vi "WinCI Get Advanced Command Options.vi"(7 "advanced options in":variant, 8 "error in (no error)":errorcluster, 10 "command":T1 items=["GET", "CHECKOUT", "CHECKIN", "UNDOCHECKOUT", "ADD", "REMOVE", "COMPARE", "FILEHISTORY", "FILEPROPERTIES", "CONFIGOPTIONS"], 11 "source control reference in":T2) -> (0 "error out":errorcluster, 1 "dialog box cancelled?":bool, 2 "status message":string, 3 "source control reference out":T2, 5 "advanced options out":variant)   [LabVIEW 2020, in "NI_SCC_WinCI.lvlib"]
uses:
  <vilib>/SourceControl/Providers/WinCI/NI_SCC_WinCI.lvlib
  <vilib>/SourceControl/sccapi/SCCAPI Refnum.ctl
  <vilib>/SourceControl/sccapi/SCCAPI Command.ctl
  <vilib>/SourceControl/support/SCCSup Message Strings GLBL.vi
  <vilib>/SourceControl/sccapi/NI_SCC.lvlib
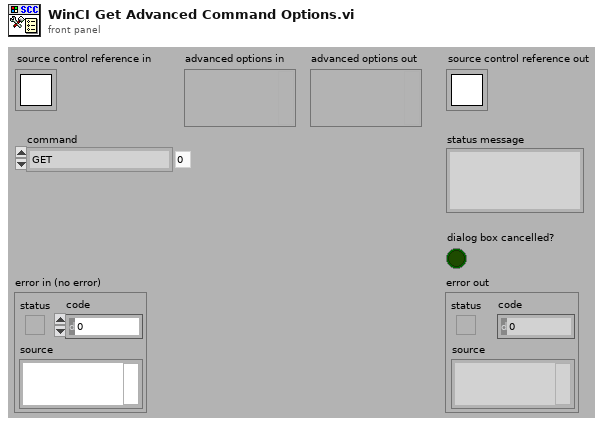
[diagram p1: front panel]
types:
  T1 = typedef "NI_SCC.lvlib/SCCAPI Command.ctl" = i32
  T2 = typedef "NI_SCC.lvlib/SCCAPI Refnum.ctl" = refnum<k1>
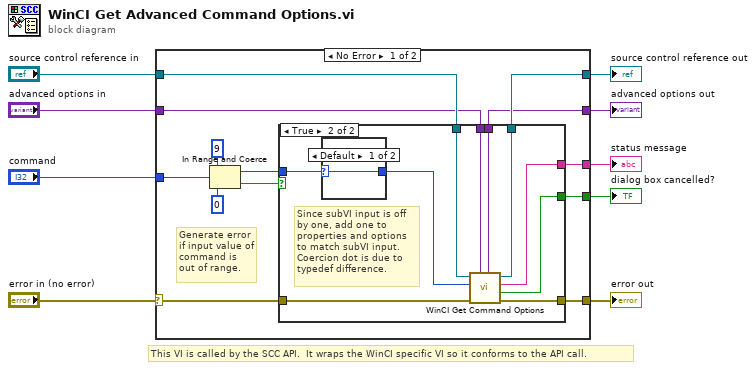
[diagram p0: block diagram]
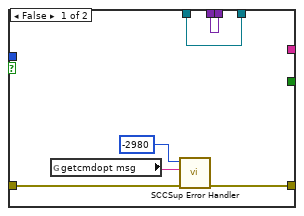
[diagram p2: hidden frame]
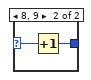
[diagram p3: hidden frame]
diagram:
  # "This VI is called by the SCC API.  It wraps the WinCI specific VI so it conforms to the API call."
  n1 = case shown="No Error" "error in (no error)" {
    selector: "error in (no error)" -> [w19 w44]
    tunnel: [w18 w44] -> w8
    tunnel: "source control reference in" -> [w17 w43]
    tunnel: [w15 _] -> w6
    tunnel: "command" -> [w20 _]
    tunnel: [w14 _] -> w4
    tunnel: [w16 w43] -> w3
    tunnel: [w12 w42] -> w2
    tunnel: "advanced options in" -> [w11 w42]
    frame No Error {
      # "Generate error if input value of command is out of range."
      n2 = In Range and Coerce(upper limit=9, x=w20, lower limit=0) -> (coerced(x)=w13:T1, In Range?=w10:bool)
      n3 = case shown="True" w10 {
        tunnel: w19 -> [w25 w29]
        tunnel: [w24 w30] -> w18
        tunnel: w17 -> [w27 w34]
        tunnel: [w27 w35] -> w16
        tunnel: [_ w32] -> w15
        tunnel: [_ w31] -> w14
        tunnel: w13 -> [_ w38]
        tunnel: [w28 w36] -> w12
        tunnel: w11 -> [w28 w37]
        frame False {
          n4 = global read "SCCSup Message Strings GLBL.vi" "getcmdopt msg"() -> (w26:string)
          n5 = call <vilib>:"SCCSup Error Handler.vi"("error in (no error)"=w25, "operation message"=w26, "scc error code"=-2980 ("error code")) -> ("error out"=w24:errorcluster)  [unwired: 1 in, 7 out]
        }
        frame True {
          # "Since subVI input is off by one, add one to properties and options to match subVI input.  Coercion dot is due to typedef difference."
          n6 = case shown="Default" w38 {
            selector: w38 -> [w39 w41]
            tunnel: [w39 w40] -> w33
            frame Default {
            }
            frame 8, 9 {
              n7 = Increment(x=w41) -> (x+1=w40:T1)
            }
          }
          n8 = call <vilib>:"WinCI Get Command Options.vi"("advanced options in"=w37, "error in (no error)"=w29, "interface command"=w33, "source control reference in"=w34) -> ("error out"=w30:errorcluster, "dialog box cancelled?"=w31:bool, "status message"=w32:string, "source control reference out"=w35:T2, "advanced options out"=w36:variant)  [unwired: 3 out]
        }
      }
    }
    frame Error {
    }
  }
  "error out" <- w8
  "status message" <- w6
  "source control reference out" <- w3
  "dialog box cancelled?" <- w4
  "advanced options out" <- w2
